vi "FindDependency(byKey).vi"(8 "error in (no error)":errorcluster, 9 "Search Key (Name)":T1, 10 "Key":string, 11 "SMO in":refnum<class "SMO.lvclass">) -> (0 "error out":errorcluster, 1 "Found?":bool, 2 "Dependency":refnum<class "SMO.lvclass">, 3 "SMO dup":refnum<class "SMO.lvclass">)   [LabVIEW 2021, in "smo.lvlib" / "SMO.lvclass"]
uses:
  SMO.lvclass
  Typedefs/Search Key.ctl
  SMO.lvclass/SMO.ctl
  Support/Attribute.Identity/Attribute.Identity.lvclass/Attribute.Identity.ctl
  Support/Attribute.Dependencies/Attribute.Dependencies.lvclass/Attribute.Dependencies.ctl
  Support/Attribute.Dependencies/List Dependencies.vi
  Private/GetVariant(Attr).vi
  Support/Attribute.Identity/Read UniqueName.vi
  Support/Attribute.Identity/Read Given Name.vi
  Support/Attribute.Identity/Read ProspectiveOwner.vi
  Private/ReftoDVR--SMO.vi
  Support/Attribute.Dependencies/Get GUIDs.vi
  Support/Attribute.Dependencies/Attribute.Dependencies.lvclass
  Support/Attribute.Identity/Attribute.Identity.lvclass
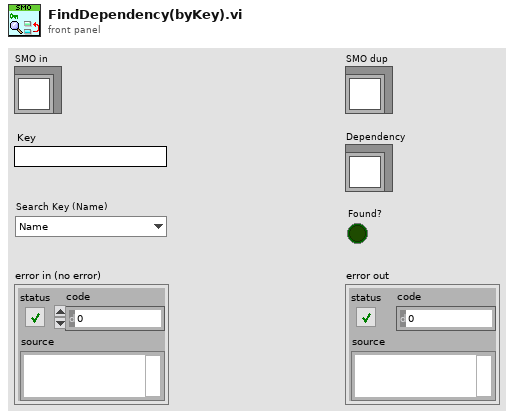
[diagram p1: front panel]
types:
  T1 = typedef "smo.lvlib/SMO.lvclass/Search Key.ctl" = enum16{"Name", "GUID", "Qualified Name", "Subsystem Path", "Configuration Path"}
  T2 = typedef "smo.lvlib/Attribute.Dependencies.lvclass/DependencyAttr--Cluster.ctl" = cluster{"Name":string, "GUID":string, "owned":bool, "shared":bool, "Level":string, "SMO":refnum<class "SMO.lvclass">}
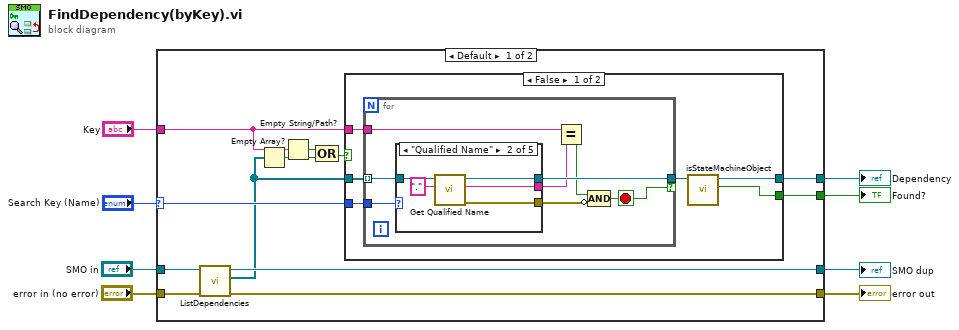
[diagram p0: block diagram]
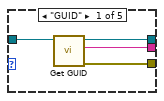
[diagram p2: hidden frame]
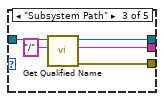
[diagram p3: hidden frame]
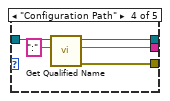
[diagram p4: hidden frame]
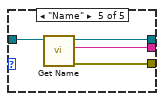
[diagram p5: hidden frame]
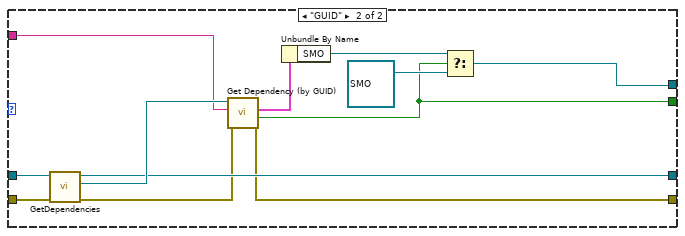
[diagram p7: hidden frame]
diagram:
  n1 = case shown="Default" "Search Key (Name)" {
    selector: "Search Key (Name)" -> [w14 _]
    tunnel: "Key" -> [w12 w67]
    tunnel: [w20 w58] -> w7
    tunnel: [w19 w64] -> w6
    tunnel: [w18 w69] -> w5
    tunnel: [w17 w61] -> w4
    tunnel: "SMO in" -> [w16 w65]
    tunnel: "error in (no error)" -> [w15 w63]
    frame Default {
      n2 = call "ListDependencies.vi"("error in (no error)"=w15, "SMO in"=w16) -> ("error out"=w20:errorcluster, "[Dependencies]"=w13:refnum<class "SMO.lvclass">[], "SMO out"=w19:refnum<class "SMO.lvclass">)  [unwired: 6 in, 1 out]
      n3 = Empty Array?(array=w13) -> (empty?=w10:bool)
      n4 = Empty String/Path?(string/path=w12) -> (empty?=w11:bool)
      n5 = Compound Arithmetic op=OR(w11, w10) -> (w9:bool)
      n6 = case shown="False" w9 {
        tunnel: [w22 _] -> w18
        tunnel: [w23 _] -> w17
        tunnel: w14 -> [w26 _]
        tunnel: w13 -> [w25 _]
        tunnel: w12 -> [w24 _]
        frame False {
          n7 = for {
            tunnel: w25 -> [w34] mode=indexing
            tunnel: [w33] -> w21 if=w28
            tunnel: w24 -> [w31]
            tunnel: w26 -> [w30]
            stop <- w28 stop-if-true
            n8 = case shown="\"Qualified Name\"" w30 {
              tunnel: w34 -> [w38 w43 w48 w53 w57]
              tunnel: [w37 w42 w47 w52 w56] -> w33
              tunnel: [w36 w41 w46 w51 w55] -> w32
              tunnel: [w35 w40 w45 w50 w54] -> w29
              frame "GUID" {
                n9 = call "Get GUID.vi"("SMO"=w38) -> ("error out"=w35:errorcluster, "GUID"=w36:string, "SMO out"=w37:refnum<class "SMO.lvclass">)  [unwired: 8 in]
              }
              frame "Qualified Name" {
                n10 = call "Get Qualified Name.vi"("separator (dot)"=".", "SMO"=w43) -> ("error out"=w40:errorcluster, "Qualified Name"=w41:string, "SMO out"=w42:refnum<class "SMO.lvclass">)  [unwired: 6 in, 1 out]
              }
              frame "Subsystem Path" {
                n11 = call "Get Qualified Name.vi"("separator (dot)"="/", "SMO"=w48) -> ("error out"=w45:errorcluster, "Qualified Name"=w46:string, "SMO out"=w47:refnum<class "SMO.lvclass">)  [unwired: 6 in, 1 out]
              }
              frame "Configuration Path" {
                n12 = call "Get Qualified Name.vi"("separator (dot)"=":", "SMO"=w53) -> ("error out"=w50:errorcluster, "Qualified Name"=w51:string, "SMO out"=w52:refnum<class "SMO.lvclass">)  [unwired: 6 in, 1 out]
              }
              frame "Name" {
                n13 = call "Get Name.vi"("SMO"=w57) -> ("error out"=w54:errorcluster, "Name"=w55:string, "SMO out"=w56:refnum<class "SMO.lvclass">)  [unwired: 6 in, 2 out]
              }
            }
            n14 = Equal?(x=w31, y=w32) -> (x = y?=w27:bool)
            n15 = Compound Arithmetic op=AND(w27, invert w29) -> (w28:bool)
          }
          n16 = call "isStateMachineObject.vi"("SMO"=w21) -> ("is SMO?"=w23:bool, "SMO out"=w22:refnum<class "SMO.lvclass">)  [unwired: 8 in, 1 out]
        }
        frame True {
        }
      }
    }
    frame "GUID" {
      n17 = call "GetDependencies.vi"("error in (no error)"=w63, "SMO in"=w65) -> ("error out"=w59:errorcluster, "Dependencies"=w68:refnum<class "Attribute.Dependencies.lvclass">, "SMO out"=w64:refnum<class "SMO.lvclass">)  [unwired: 7 in]
      n18 = call "Get Dependency (by GUID).vi"("error in (no error)"=w59, "GUID"=w67, "Attribute.Dependencies in"=w68) -> ("error out"=w58:errorcluster, "found"=w61:bool, "Dependency"=w66:T2)  [unwired: 5 in, 1 out]
      n19 = Unbundle By Name(w66) -> ("SMO"=w60:refnum<class "SMO.lvclass">)
      n20 = Select(t=w60, s=w61, f=refnum<class "SMO.lvclass"> refnum) -> (s? t:f=w69:refnum<class "SMO.lvclass">)
    }
  }
  "SMO dup" <- w6
  "error out" <- w7
  "Dependency" <- w5
  "Found?" <- w4
